vi "5.Descreate LED_0.vi"() -> ()   [LabVIEW 2015]
uses:
  <vilib>/myRIO/Instrument Drivers/Onboard IO/DIO/vis/Write.vi
  <vilib>/myRIO/Common/Instrument Driver Framework/myRIO v1.0/UART/vis/myRIO v1.0 Close UART.vi
  <vilib>/myRIO/Instrument Drivers/Onboard IO/DIO/vis/Smart Open.vi
  <vilib>/Utility/error.llb/Error Cluster From Error Code.vi
  <vilib>/myRIO/Common/Instrument Driver Framework/myRIO v1.0/DIO/vis/myRIO v1.0 Write DIO.vi
  <vilib>/myRIO/Common/Instrument Driver Framework/Utilities/vis/FPGA Ref Manager.vi
  <vilib>/myRIO/Common/Instrument Driver Framework/myRIO v1.0/myRIO v1.0 Reset FPGA.vi
  <vilib>/myRIO/Common/Instrument Driver Framework/myRIO v1.0/IRQ/vis/myRIO v1.0 IRQ Info FGV.vi
  <vilib>/myRIO/Common/Instrument Driver Framework/myRIO v1.0/IRQ/vis/myRIO v1.0 Timer IRQ Info FGV.vi
  <vilib>/myRIO/Common/Instrument Driver Framework/myRIO v1.0/IRQ/vis/myRIO v1.0 ISR Agent.vi
  <vilib>/myRIO/Instrument Drivers/Utilities/Utilities.lvlib
panel:
  in  "Tab Control":enum32{"Page 1", "Page 2"}(tab)
  in  "digital level":bool
  in  "enable blinker":bool=TRUE
  out "digital output state":bool
  in  "]":bool
  # "Descreate LED"
  # "Pardeep kumar"
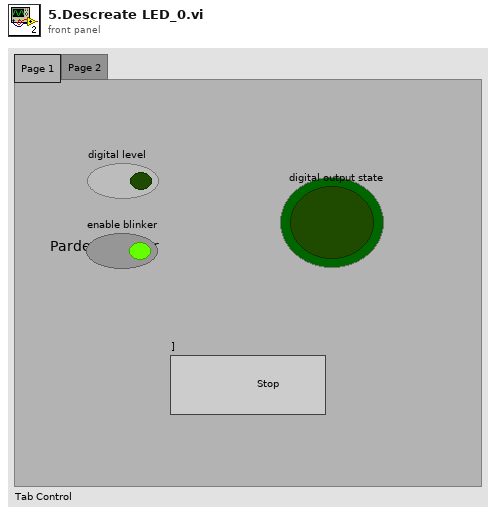
[diagram p1: front panel]
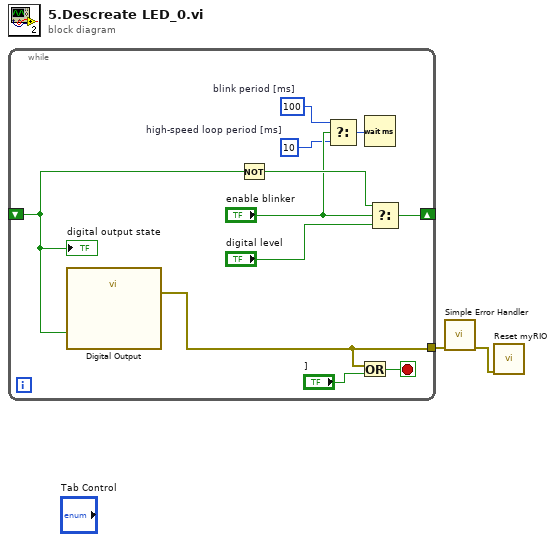
[diagram p0: block diagram]
diagram:
  n1 = while {
    tunnel: [w3] -> w2
    shift-right: [w9] -> _
    shift-left: _ -> [w11]
    stop <- w13 stop-if-true
    w4 = u32 10  # high-speed loop period [ms]
    w5 = u32 100  # blink period [ms]
    n2 = call "Digital Output"("B/DIO0 (Pin 11)"=w11) -> ("error out"=w3:errorcluster)  [unwired: 26 in]
    n3 = Not(x=w11) -> (.not. x?=w10:bool)
    n4 = Select(t=w5, s="enable blinker", f=w4) -> (s? t:f=w7:u32)
    n5 = Or(x=w3, y="]") -> (x .or. y?=w13:bool)
    n6 = Wait (ms)(milliseconds to wait=w7) -> ()  [unwired: 1 out]
    n7 = Select(t=w10, s="enable blinker", f="digital level") -> (s? t:f=w9:bool)
    "digital output state" <- w11
  }
  n8 = call <vilib>:"Simple Error Handler.vi"("error in (no error)"=w2) -> ("error out"=w1:errorcluster)  [unwired: 4 in, 4 out]
  n9 = call <vilib>:"Reset myRIO.vi"("error in (no error)"=w1) -> ()  [unwired: 10 in, 1 out]
